vi "RandDBL.vi"(3 "Limit b":dbl=1.0 caption="Limit b (1)", 5 "Limit a":dbl caption="Limit a (0)") -> (1 "Random number":dbl)   [LabVIEW 2017, in "GPNumeric.lvlib"]
doc: "Produces a <B>Random number</B> between <B>Limit a</B> and <B>Limit b</B>.\n\nIt doesn't matter which of <B>Limit a</B> and <B>Limit b</B> is highest, only the range is considered. For floating point numbers the lowest limit is included in the range of random numbers, the highest limit is not.\n\nIf either limit is +/-infinity or NaN, the output will be NaN.\n\nThis VI is polymorphic, right click on it to select the data type.\n\nThis VI is inlined.\n\nSteen Schmidt\nGPower\n5/4 2014"
uses:
  GPNumeric.lvlib
panel:
  # "Copyright © 2014\nGPower\nSee enclosed license file for terms and conditions"
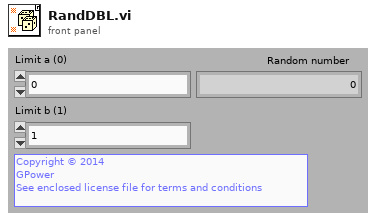
[diagram p1: front panel]
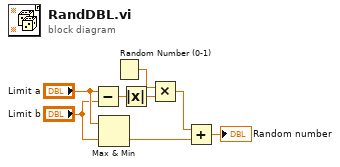
[diagram p0: block diagram]
diagram:
  n1 = Subtract(x="Limit a", y="Limit b") -> (x-y=w8:dbl)
  n2 = Max & Min(x="Limit a", y="Limit b") -> (min(x,y)=w7:dbl)  [unwired: 1 out]
  n3 = Random Number (0-1)() -> (number: 0 to 1=w1:dbl)
  n4 = Absolute Value(x=w8) -> (abs(x)=w3:dbl)
  n5 = Multiply(x=w1, y=w3) -> (x*y=w2:dbl)
  n6 = Add(x=w2, y=w7) -> (x+y=→"Random number":dbl)
